vi "nuovo progressivo.vi"(8 "anno":string, 9 "banco":string, 10 "table":string, 11 "Refnum in":T1) -> (2 "progressivo":string, 3 "Refnum out":T1)   [LabVIEW 2019]
uses:
  <vilib>/addons/database/Connection.llb/Conn ObjectReference.ctl
  <vilib>/addons/database/NI_Database_API.lvlib
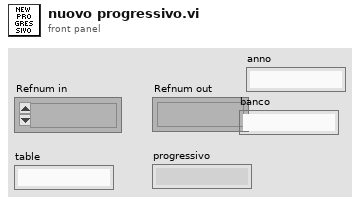
[diagram p1: front panel]
types:
  T1 = typedef "NI_Database_API.lvlib/Conn ObjectReference.ctl" = refnum<k1>
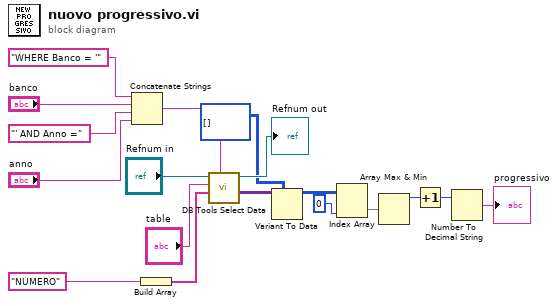
[diagram p0: block diagram]
diagram:
  n1 = Concatenate Strings("WHERE Banco = '", "banco", "' AND Anno =" ("string"), "anno") -> (w1:string)
  n2 = Build Array("NUMERO" ("SQL query")) -> (w8:string[])
  n3 = call <vilib>:"DB Tools Select Data.vi"("condition"=w1, "columns"=w8, "table"="table", "connection reference"="Refnum in") -> ("data"=w9:variant[][], "connection reference out"=→"Refnum out":T1)  [unwired: 2 in, 1 out]
  n4 = Variant To Data(type=i32[][] [], Variant=w9) -> (data=w11:i32[][])  [unwired: 1 in, 1 out]
  n5 = Index Array(array=w11, index (col)=0 ("disabled index (col)")) -> (element=w13:i32[])  [unwired: 1 in]
  n6 = Array Max & Min(array=w13) -> (max value=w14:i32)  [unwired: 3 out]
  n7 = Increment(x=w14) -> (x+1=w15:i32)
  n8 = Number To Decimal String(number=w15) -> (decimal integer string=→"progressivo":string)  [unwired: 1 in]
